vi "求最大值.vi"() -> ()   [LabVIEW 2010]
panel:
  in  "循环次数":i32=20
  out "最大值":dbl format="%.2f"
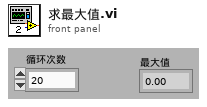
[diagram p1: front panel]
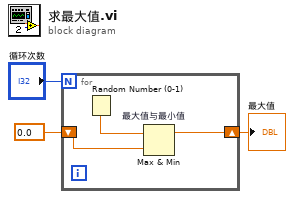
[diagram p0: block diagram]
diagram:
  n1 = for {
    N: "循环次数" -> [_]
    shift-right: [w4] -> w3
    shift-left: 0.0 -> [w5]
    n2 = Random Number (0-1)() -> (number: 0 to 1=w6:dbl)
    n3 = Max & Min "最大值与最小值"(x=w6, y=w5) -> (max(x,y)=w4:dbl)  [unwired: 1 out]
  }
  "最大值" <- w3
